vi "main.vi"() -> ()   [LabVIEW 2023]
uses:
  CONTROLS/States.ctl
panel:
  out "Meldung":string
  out "Enum":T1
  in  "stop":bool
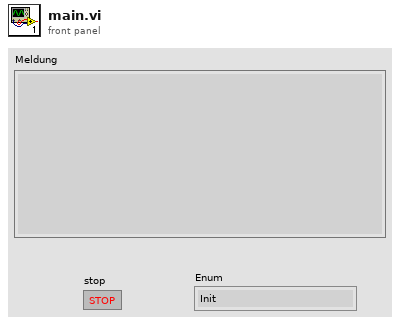
[diagram p1: front panel]
types:
  T1 = typedef "States.ctl" = enum16{"Init", "read", "write", "Kundeneingabe", "Betonauswahl", "Bezahlprozess", "Rechnung", "Zutaten mit Gewichtmessung", "Stop"}
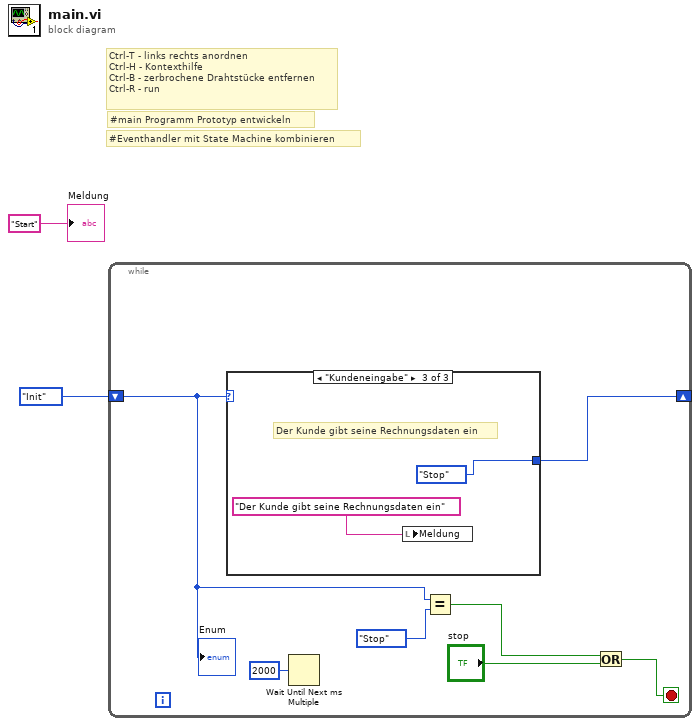
[diagram p0: block diagram]
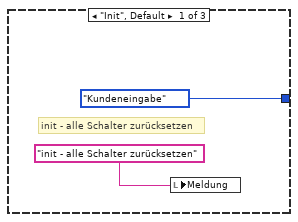
[diagram p2: hidden frame]
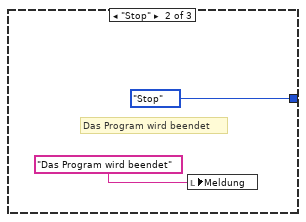
[diagram p3: hidden frame]
diagram:
  # "#Eventhandler mit State Machine kombinieren"
  # "#main Programm Prototyp entwickeln"
  # "Ctrl-T - links rechts anordnen\nCtrl-H - Kontexthilfe\nCtrl-B - zerbrochene Drahtstücke entfernen\nCtrl-R - run"
  n1 = while {
    shift-right: [w9] -> _
    shift-left: States."Init" -> [w8]
    stop <- w4 stop-if-true
    n2 = case shown="\"Kundeneingabe\"" w8 {
      tunnel: [States."Kundeneingabe" States."Stop" States."Stop"] -> w9
      frame "Init", Default {
        # "init - alle Schalter zurücksetzen"
        n3 = local write "Meldung"("init - alle Schalter zurücksetzen" ("Meldung")) -> ()
      }
      frame "Stop" {
        # "Das Program wird beendet"
        n4 = local write "Meldung"("Das Program wird beendet" ("Meldung")) -> ()
      }
      frame "Kundeneingabe" {
        # "Der Kunde gibt seine Rechnungsdaten ein"
        n5 = local write "Meldung"("Der Kunde gibt seine Rechnungsdaten ein" ("Meldung")) -> ()
      }
    }
    n6 = Wait Until Next ms Multiple(millisecond multiple=u32 2000) -> ()  [unwired: 1 out]
    n7 = Equal?(x=w8, y=States."Stop") -> (x = y?=w6:bool)
    n8 = Or(x=w6, y="stop") -> (x .or. y?=w4:bool)
    "Enum" <- w8
  }
  "Meldung" <- "Start" ("Meldung")
